vi "Set Cobra Data.vi"(8 "error in (no error)":errorcluster, 10 "Run":bool=TRUE, 11 "Test in":refnum<class "Test.lvclass">) -> (0 "error out":errorcluster, 3 "Test out":refnum<class "Test.lvclass">)   [LabVIEW 2019, in "Test.lvlib" / "Test.lvclass"]
uses:
  Test.lvclass
  Test.lvclass/Test.ctl
  Platform/Platform Messages/Get Instrument Dataset Msg/Get Instrument Data Msg.lvclass/Get Instrument Data Msg.ctl
  <vilib>/ActorFramework/Message Enqueuer/Message Enqueuer.lvclass/Message Enqueuer.ctl
  <vilib>/ActorFramework/Message Enqueuer/Enqueue.vi
  Platform/Platform Messages/Get Instrument Dataset Msg/Get Instrument Data Msg.lvclass
  C:/Program Files (x86)/National Instruments/LabVIEW 2019/vi.lib/ActorFramework/Message/Message.lvclass
  <vilib>/ActorFramework/Message Priority Queue/Priority Enqueue.vi
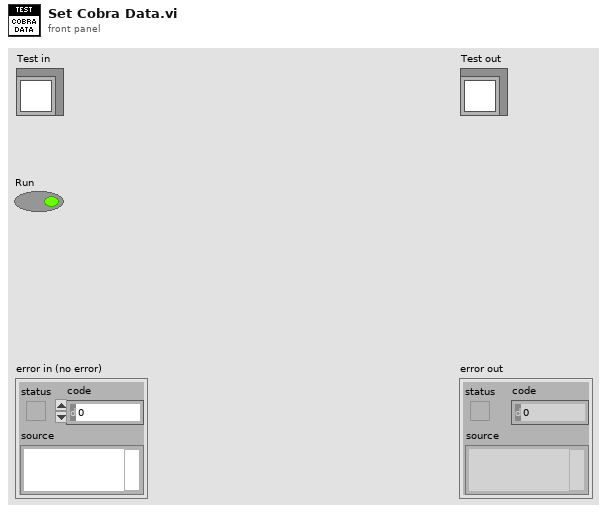
[diagram p1: front panel]
types:
  T1 = map{string, cluster{"Selected Heads":string, "Instrument":refnum<class "Message Enqueuer.lvclass">, "Platform":refnum<class "Message Enqueuer.lvclass">}}
  T2 = typedef "Test.lvlib/Cobra Data.ctl" = cluster{"M2 Dataset":cluster{"Read Temp":dbl, "Feedback":u8, "Set Temp":dbl}, "M1 Dataset":cluster{"Read Temp":dbl, "Feedback":u8, "Set Temp":dbl}, "Comp":bool}
  T3 = cluster{"Selected Heads":string, "Instrument":refnum<class "Message Enqueuer.lvclass">, "Platform":refnum<class "Message Enqueuer.lvclass">}
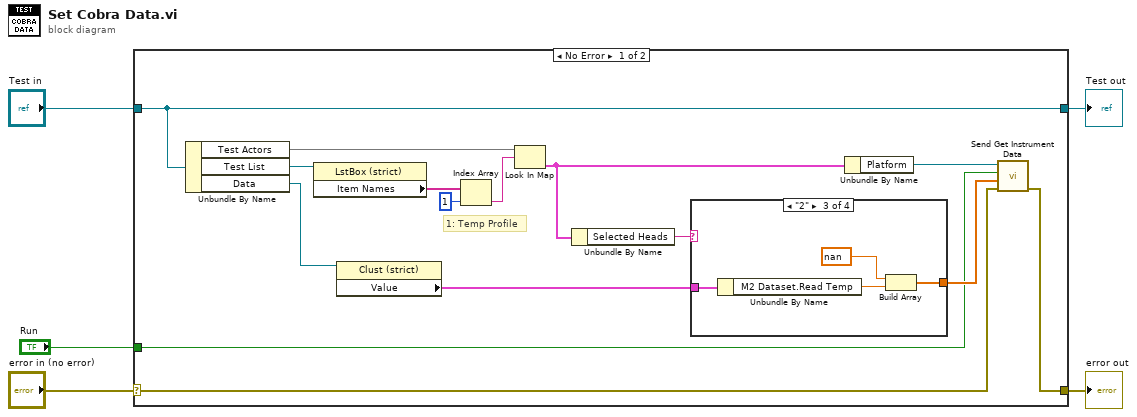
[diagram p0: block diagram]
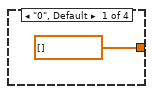
[diagram p2: hidden frame]
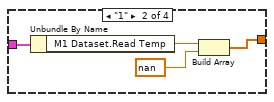
[diagram p3: hidden frame]
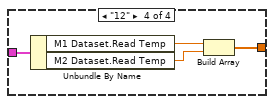
[diagram p4: hidden frame]
diagram:
  n1 = case shown="No Error" "error in (no error)" {
    selector: "error in (no error)" -> [w8 w35]
    tunnel: [w7 w35] -> w4
    tunnel: [w11 w34] -> w2
    tunnel: "Test in" -> [w11 w34]
    tunnel: "Run" -> [w6 _]
    frame No Error {
      # "1: Temp Profile"
      n2 = Unbundle By Name(w11) -> ("Test Actors"=w14:T1, "Test List"=w13:refnum<vi>, "Data"=w17:refnum<vi>)
      n3 = property class="LstBox (strict)"(reference=w13) -> ("Item Names"=w12:string[])  [unwired: 1 in, 2 out]
      n4 = property class="Clust (strict)"(reference=w17) -> ("Value"=w16:T2)  [unwired: 1 in, 2 out]
      n5 = Index Array(array=w12, index=1) -> (element=w15:string)
      n6 = Look In Map(map=w14, key=w15) -> (value=w18:T3)  [unwired: 1 in, 1 out]
      n7 = Unbundle By Name(w18) -> ("Selected Heads"=w19:string)
      n8 = case shown="\"2\"" w19 {
        tunnel: w16 -> [_ w25 w29 w33]
        tunnel: [dbl[] [] w23 w27 w31] -> w9
        frame "0", Default {
        }
        frame "1" {
          n9 = Unbundle By Name(w25) -> ("M1 Dataset.Read Temp"=w24:dbl)
          n10 = Build Array(w24, nan) -> (w23:dbl[])
        }
        frame "2" {
          n11 = Unbundle By Name(w29) -> ("M2 Dataset.Read Temp"=w28:dbl)
          n12 = Build Array(nan, w28) -> (w27:dbl[])
        }
        frame "12" {
          n13 = Unbundle By Name(w33) -> ("M1 Dataset.Read Temp"=w30:dbl, "M2 Dataset.Read Temp"=w32:dbl)
          n14 = Build Array(w30, w32) -> (w31:dbl[])
        }
      }
      n15 = Unbundle By Name(w18) -> ("Platform"=w10:refnum<class "Message Enqueuer.lvclass">)
      n16 = call "Send Get Instrument Data.vi"("error in (no error)"=w8, "Data"=w9, "Connection"=w6, "Message Enqueuer"=w10) -> ("error out"=w7:errorcluster)  [unwired: 6 in, 1 out]
    }
    frame Error {
    }
  }
  "error out" <- w4
  "Test out" <- w2
